vi "Stage Global.vi"() -> ()   [LabVIEW 2012]
panel:
  in  "Position":dbl
  out "Speed":dbl
  out "Initial Position":dbl
  out "Final Position":dbl
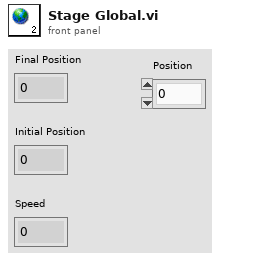
[diagram p1: front panel]
diagram:
